vi "Determine Clicked Array Element Index - Calculate Gapped and Un-Gapped Coordinates.vi"(0 "Array Reference":refnum<vi>, 2 "Array Min Properties.Position.Left":i32, 3 "Array Min Properties.Position.Top":i32, 5 "error in (no error)":errorcluster, 6 "Select Item":T1(ring)) -> (14 "dup Array Reference":refnum<vi>, 17 "Un-gapped coordinates":i32[](array[numeric]), 18 "Gapped coordinates":i32[](array[numeric]), 19 "error out":errorcluster)   [LabVIEW 2021, in "Arrays.lvlib"]
doc: "Determine Clicked Array Element Index - Calculate Gapped and Un-Gapped Coordinates.vi\n\nDescription:\nThis VI calculates the top or left array element coordinates (gapped and un-gapped) based on the setting of the Select Item input.\n\nInputs:\nArray Reference - Reference to the array to operate on.\n\nSelect Item - Specifies the coordinates (Row or Column) to calculate.\n\nArray Min Properties.Position.Left - The left position of the array when the scrollbars, index display, label and caption are hidden.\n\nArray Min Properties.Position.Top - The top position of the array when the scrollbars, index display, label and caption are hidden.\n\nerror in - Standard error cluster.\n\nOutputs:\ndup Array Reference - Dup reference to the array to operate on.\n\nUn-gapped coordinates - The calculated un-gapped coordinates.\n\nGapped coordinates - The calculated gapped coordinates.\n\nerror out - Standard error cluster.\n\nDeveloped By:\nMark.ridgley\nMark.Ridgley_LabVIEW.Developer@comcast.net"
uses:
  Arrays.lvlib
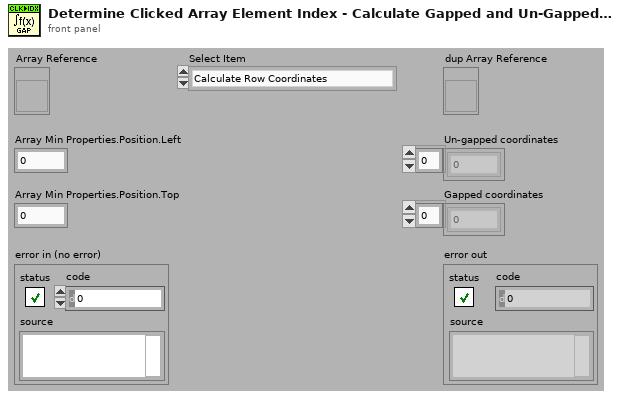
[diagram p1: front panel]
types:
  T1 = enum16{"Calculate Row Coordinates", "Calculate Col Coordinates"}
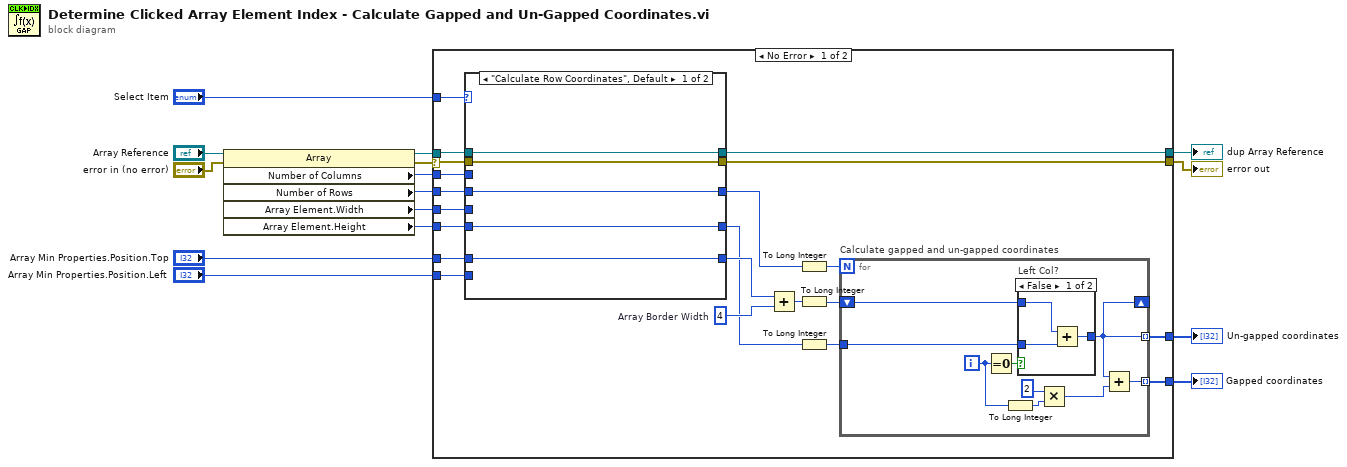
[diagram p0: block diagram]
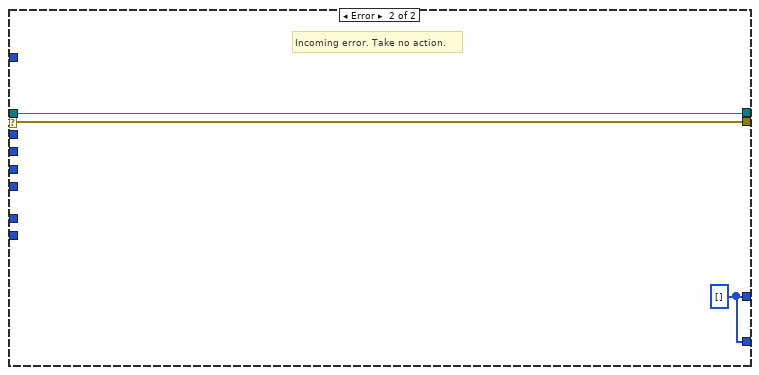
[diagram p4: hidden frame]
diagram:
  n1 = property class="Array"(reference="Array Reference", error in="error in (no error)") -> (reference out=w7:refnum<vi>, error out=w5:errorcluster, "Number of Columns"=w4:u32, "Number of Rows"=w3:u32, "Array Element.Width"=w2:u32, "Array Element.Height"=w1:u32)
  n2 = case shown="No Error" w5 {
    selector: w5 -> [w24 w62]
    tunnel: [w36 w60] -> w15
    tunnel: [w35 w60] -> w14
    tunnel: "Select Item" -> [w32 _]
    tunnel: "Array Min Properties.Position.Left" -> [w30 _]
    tunnel: "Array Min Properties.Position.Top" -> [w28 _]
    tunnel: w7 -> [w25 w61]
    tunnel: [w27 w62] -> w9
    tunnel: [w26 w61] -> w10
    tunnel: w4 -> [w23 _]
    tunnel: w3 -> [w22 _]
    tunnel: w2 -> [w21 _]
    tunnel: w1 -> [w20 _]
    frame No Error {
      w19 = 4  # Array Border Width
      n3 = case shown="\"Calculate Row Coordinates\", Default" w32 {
        tunnel: w23 -> [_ w46]
        tunnel: [w41 w46] -> w31
        tunnel: w30 -> [_ w45]
        tunnel: [w40 w45] -> w29
        tunnel: w22 -> [w41 _]
        tunnel: w28 -> [w40 _]
        tunnel: w24 -> [w39 w43]
        tunnel: w25 -> [w38 w44]
        tunnel: [w39 w43] -> w27
        tunnel: [w38 w44] -> w26
        tunnel: w21 -> [_ w42]
        tunnel: [w37 w42] -> w18
        tunnel: w20 -> [w37 _]
        frame "Calculate Row Coordinates", Default {
        }
        frame "Calculate Col Coordinates" {
        }
      }
      n4 = Add(x=w29, y=w19) -> (x+y=w34:i32)
      n5 = To Long Integer(number=w31) -> (32bit integer=w33:i32)
      n6 = To Long Integer(number=w34) -> (32bit integer=w17:i32)
      n7 = To Long Integer(number=w18) -> (32bit integer=w16:i32)
      n8 = for "Calculate gapped and un-gapped coordinates" {
        N: w33 -> [_]
        tunnel: w16 -> [w53]
        tunnel: [w51] -> w36 mode=indexing
        shift-right: [w51] -> _
        shift-left: w17 -> [w55]
        tunnel: [w49] -> w35 mode=indexing
        i -> [w50]
        n9 = Equal To 0?(x=w50) -> (x = 0?=w54:bool)
        n10 = To Long Integer(number=w50) -> (32bit integer=w47:i32)
        n11 = case "Left Col?" shown="False" w54 {
          tunnel: w55 -> [w58 w59]
          tunnel: [w57 w59] -> w51
          tunnel: w53 -> [w56 _]
          frame False {
            n12 = Add(x=w58, y=w56) -> (x+y=w57:i32)
          }
          frame True {
          }
        }
        n13 = Multiply(x=2, y=w47) -> (x*y=w48:i32)
        n14 = Add(x=w51, y=w48) -> (x+y=w49:i32)
      }
    }
    frame Error {
      w60 = i32[] []
      # "Incoming error. Take no action."
    }
  }
  "Un-gapped coordinates" <- w15
  "Gapped coordinates" <- w14
  "dup Array Reference" <- w10
  "error out" <- w9
